vi "while.vi"() -> ()   [LabVIEW 2020]
panel:
  out "Array":dbl[](array[numeric])
  out "Numeric 2":dbl
  out "Numeric":dbl
  in  "stop":bool
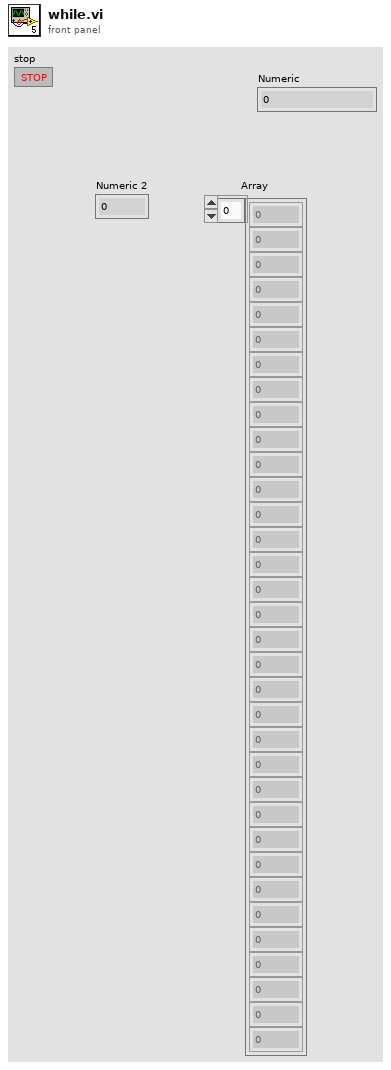
[diagram p1: front panel]
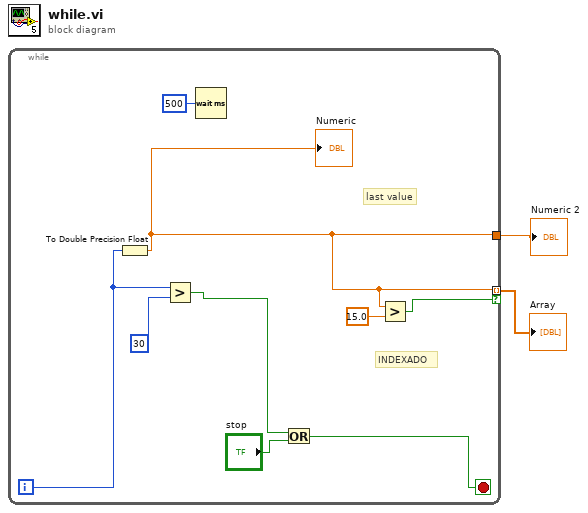
[diagram p0: block diagram]
diagram:
  n1 = while {
    tunnel: [w4] -> w2
    tunnel: [w4] -> w1 mode=indexing if=w5
    i -> [w7]
    stop <- w9 stop-if-true
    # "INDEXADO"
    # "last value"
    n2 = To Double Precision Float(number=w7) -> (double precision float=w4:dbl)
    "Numeric" <- w4
    n3 = Greater?(x=w7, y=30) -> (0:w6:bool)
    n4 = Wait (ms)(milliseconds to wait=u32 500) -> ()  [unwired: 1 out]
    n5 = Or(x=w6, y="stop") -> (x .or. y?=w9:bool)
    n6 = Greater?(x=w4, y=15.0) -> (0:w5:bool)
  }
  "Numeric 2" <- w2
  "Array" <- w1
